vi "WFS Get Master Gain Range.vi"(8 "error in (no error)":errorcluster {"code" format="%.0x"}, 11 "instrument handle":refnum<visa-resource-name>) -> (0 "error out":errorcluster {"code" format="%.0x"}, 1 "Master Gain Max":dbl, 2 "Master Gain Min":dbl, 3 "instrument handle out":refnum<visa-resource-name>)   [LabVIEW 2020]
doc: "This VI returns the available linear master gain range of the WFS camera.\n\nNote: Master gain increases image noise! Use higher exposure time to set the WFS camera more sensitive.\nLowest master gain of WFS10 camera is 1.5.\nMaster gain of WFS20 camera is fixed to 1.0."
uses:
  WFS_32.dll
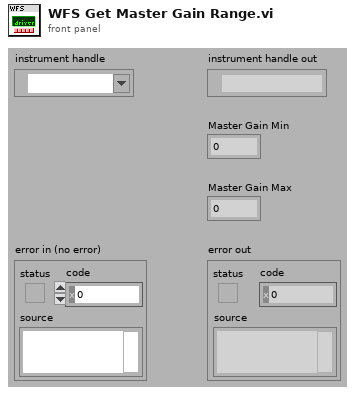
[diagram p1: front panel]
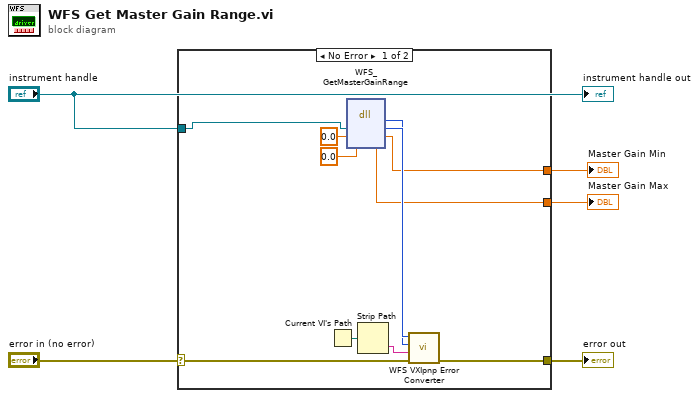
[diagram p0: block diagram]
diagram:
  n1 = case shown="No Error" "error in (no error)" {
    selector: "error in (no error)" -> [w11 w17]
    tunnel: [w10 w17] -> w5
    tunnel: "instrument handle" -> [w15 _]
    tunnel: [w8 _] -> w2
    tunnel: [w6 _] -> w1
    frame No Error {
      n2 = Current VI's Path() -> (path=w16:path)
      n3 = dll-call lib="WFS_*.*" fn="WFS_GetMasterGainRange"("Instrument Handle"=w15, "Master Gain Min"=0.0, "Master Gain Max"=0.0) -> (w13:i32, "Instrument Handle"=w14:u32, "Master Gain Min"=w8:dbl, "Master Gain Max"=w6:dbl)  [unwired: 3 in, 2 out]
      n4 = Strip Path(path=w16) -> (name=w12:string)  [unwired: 1 out]
      n5 = call "WFS VXIpnp Error Converter.vi"("error in (no error)"=w11, "Name Of VI (\"\")"=w12, "CVI Error Code (0)"=w13, "instrument handle"=w14) -> ("error out"=w10:errorcluster)  [unwired: 6 in, 1 out]
    }
    frame Error {
    }
  }
  "error out" <- w5
  "Master Gain Min" <- w2
  "Master Gain Max" <- w1
  "instrument handle out" <- "instrument handle"
